vi "Build Error FEFF Filter Query.vi"(10 "Stop Test Cycle":string(combo) caption="Test Cycle", 11 "Start Test Cycle":string(combo) caption="Test Cycle") -> (3 "String":string)   [LabVIEW 2023, in "Data Analysis.lvlib"]
uses:
  Data Analysis.lvlib
  <vilib>/Utility/error.llb/Trim Whitespace One-Sided.vi
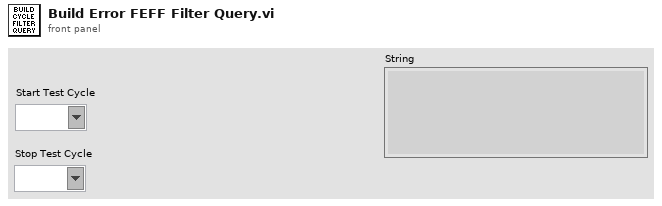
[diagram p1: front panel]
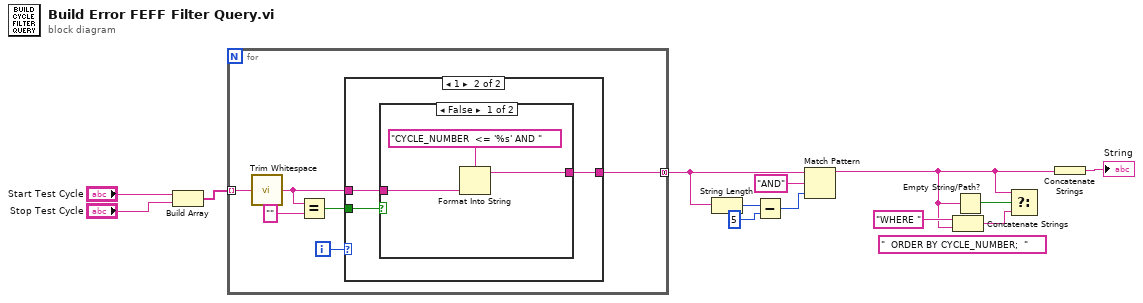
[diagram p0: block diagram]
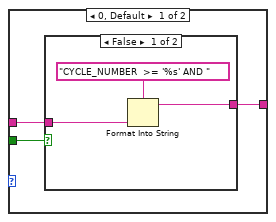
[diagram p2: hidden frame]
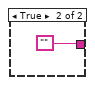
[diagram p3: hidden frame]
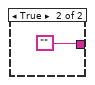
[diagram p4: hidden frame]
diagram:
  (unwired) "  ORDER BY CYCLE_NUMBER;  "
  n1 = Build Array("Start Test Cycle", "Stop Test Cycle") -> (w13:string[])
  n2 = for {
    tunnel: w13 -> [w19] mode=indexing
    tunnel: [w14] -> w7 mode=concatenating
    i -> [w17]
    n3 = call <vilib>:"Trim Whitespace.vi"("string"=w19) -> ("trimmed string"=w16:string)  [unwired: 1 in]
    n4 = Equal?(x=w16, y="") -> (x = y?=w15:bool)
    n5 = case shown="1" w17 {
      tunnel: w16 -> [w21 w28]
      tunnel: w15 -> [w22 w29]
      tunnel: [w20 w27] -> w14
      frame 0, Default {
        n6 = case shown="False" w22 {
          tunnel: w21 -> [w24 _]
          tunnel: [w23 ""] -> w20
          frame False {
            n7 = Format Into String(format string="CYCLE_NUMBER  >= '%s' AND ", w24) -> (resulting string=w23:string)  [unwired: 2 in, 1 out]
          }
          frame True {
          }
        }
      }
      frame 1 {
        n8 = case shown="False" w29 {
          tunnel: w28 -> [w31 _]
          tunnel: [w30 ""] -> w27
          frame False {
            n9 = Format Into String(format string="CYCLE_NUMBER  <= '%s' AND ", w31) -> (resulting string=w30:string)  [unwired: 2 in, 1 out]
          }
          frame True {
          }
        }
      }
    }
  }
  n10 = String Length(string=w7) -> (length=w6:i32)
  n11 = Subtract(x=w6, y=5) -> (x-y=w4:i32)
  n12 = Match Pattern(string=w7, regular expression="AND", offset (0)=w4) -> (before substring=w1:string)  [unwired: 3 out]
  n13 = Concatenate Strings("WHERE ", w1) -> (w10:string)
  n14 = Empty String/Path?(string/path=w1) -> (empty?=w12:bool)
  n15 = Select(t=w1, s=w12, f=w10) -> ()  [unwired: 1 out]
  n16 = Concatenate Strings(w1) -> (→"String":string)
